vi "ReadData.vi"(8 "error in (no error)":errorcluster, 11 "NI_DAQmx(AI) in":refnum<class "NI_DAQmx(AI).lvclass">) -> (0 "error out":errorcluster, 2 "Waveform":waveform(dbl)[](array[waveform]), 3 "NI_DAQmx(AI) out":refnum<class "NI_DAQmx(AI).lvclass">)   [LabVIEW 2025, in "NI_DAQmx(AI).lvclass"]
uses:
  NI_DAQmx(AI).lvclass
  D:/Hardware/DAQ/DAQ_Abstr/Task_Abstr/Task_Abstr/Task_Abstr.lvclass
  D:/Hardware/DAQ/DAQ_Abstr/Task_Type/AI_Task/AI_Task/AI_Task.lvclass
  D:/Hardware/DAQ/DAQ_Abstr/Task_Type/Waveform_Task/Waveform_Task/Waveform_Task.lvclass
  NI_DAQmx(AI).lvclass/NI_DAQmx(AI).ctl
  <vilib>/DAQmx/read.llb/DAQmx Read (Analog 1D Wfm NChan NSamp).vi
  Read task.vi
  <vilib>/DAQmx/miscellaneous.llb/DAQmx Fill In Error Info.vi
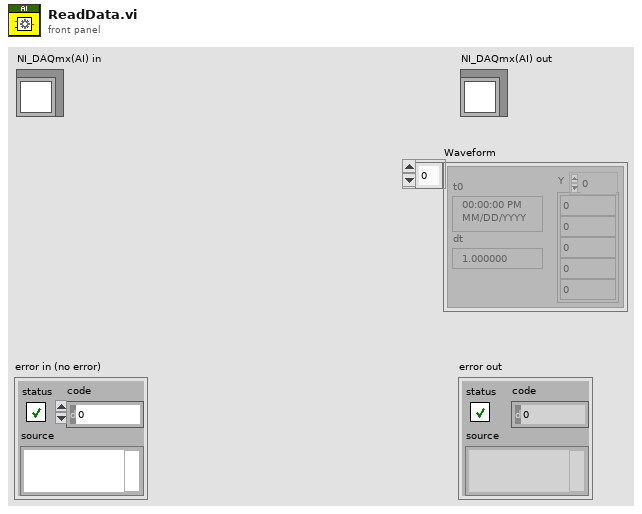
[diagram p1: front panel]
types:
  T1 = typedef "DAQ_Module.lvlib/DAQ_Module.lvclass/DAQ_Task_Config.ctl" = cluster{"Drive":T2, "TaskType":T3, "PhysicalChannels":string, "SampleRateConfiguration":T4, "ChannelConfig":map{string, cluster{"PhysicalChannels":string, "Config":string}}, "Enable":bool, "ShowPanel":bool}
  T2 = typedef "DAQ_Module.lvlib/DAQ_Module.lvclass/DAQ_HW_Type.ctl" = enum16{"NI_DAQmx", "Simulated_DAQ"}
  T3 = typedef "DAQ_Module.lvlib/DAQ_Module.lvclass/DAQ_Task_Type.ctl" = enum16{"AI", "Linear", "Angular", "AO"}
  T4 = typedef "DAQ_Module.lvlib/DAQ_Module.lvclass/DAQ_SampleRateConfig.ctl" = cluster{"SampleRate":dbl, "SamplesPerChannel":u32, "SamplesPerRead":i32, "SampleMode":i32, "Clock Source":string}
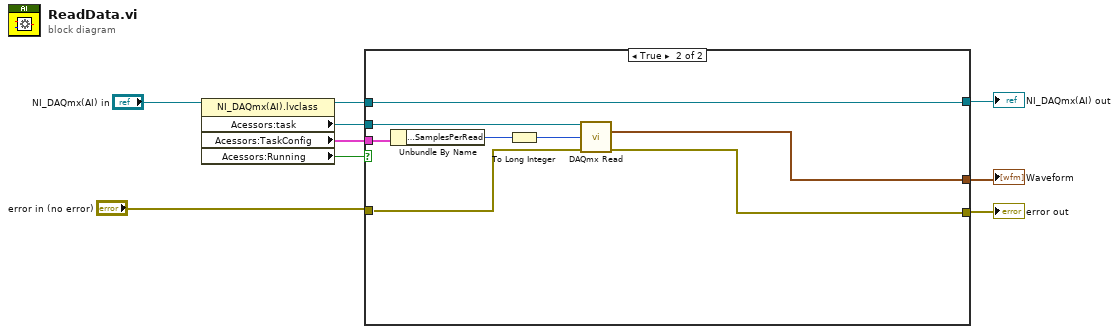
[diagram p0: block diagram]
diagram:
  n1 = property class="NI_DAQmx(AI).lvclass"(reference="NI_DAQmx(AI) in") -> (reference out=w5:refnum<class "NI_DAQmx(AI).lvclass">, "Acessors:task"=w9:refnum<k21>, "Acessors:TaskConfig"=w6:T1, "Acessors:Running"=w1:bool)  [unwired: 1 in, 1 out]
  n2 = case shown="True" w1 {
    tunnel: w9 -> [_ w19]
    tunnel: "error in (no error)" -> [w10 w18]
    tunnel: [w10 w17] -> w7
    tunnel: w6 -> [_ w16]
    tunnel: w5 -> [w11 w13]
    tunnel: [w11 w13] -> w4
    tunnel: [_ w12] -> w3
    frame False {
    }
    frame True {
      n3 = Unbundle By Name(w16) -> ("SampleRateConfiguration.SamplesPerRead"=w15:i32)
      n4 = To Long Integer(number=w15) -> (32bit integer=w14:i32)
      n5 = call-poly <vilib>:"DAQmx Read.vi"("task/channels in"=w19, "number of samples per channel"=w14, "error in"=w18) -> ("data"=w12:waveform(dbl)[], "error out"=w17:errorcluster)  [unwired: 10 in, 1 out]
    }
  }
  "error out" <- w7
  "NI_DAQmx(AI) out" <- w4
  "Waveform" <- w3
